vi "Write_All_Channels_to_Month_file.vi"(0 "Current Time":dbl, 1 "Channel Names":string[](array[string]), 2 "Channel Values":string[](array[string]), 3 "Comments":string[](array[string])) -> (7 "File Updated?":bool)   [LabVIEW 2020]
uses:
  Anemometry/Anemometry Sub Vis/Globals/Preference_global.vi
  Anemometry/Anemometry Sub Vis/Globals/Constants_global.vi
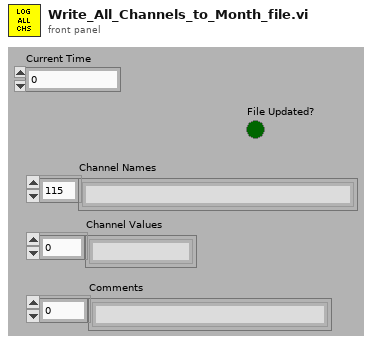
[diagram p1: front panel]
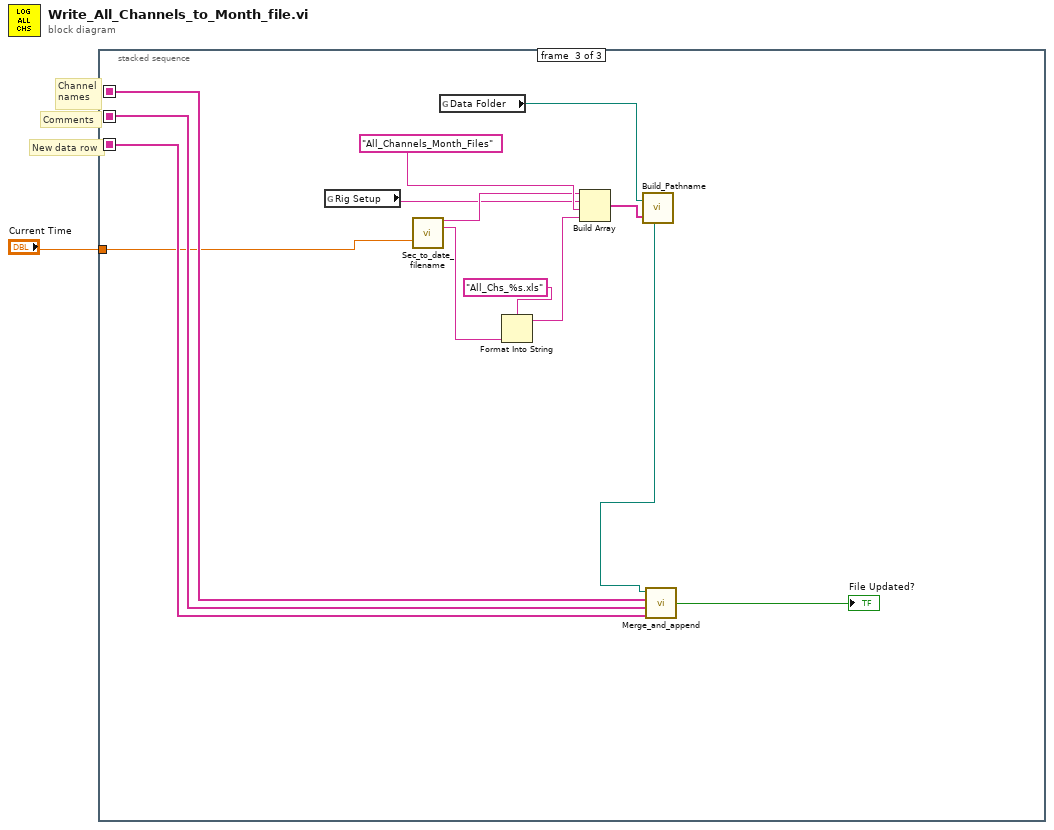
[diagram p0: block diagram]
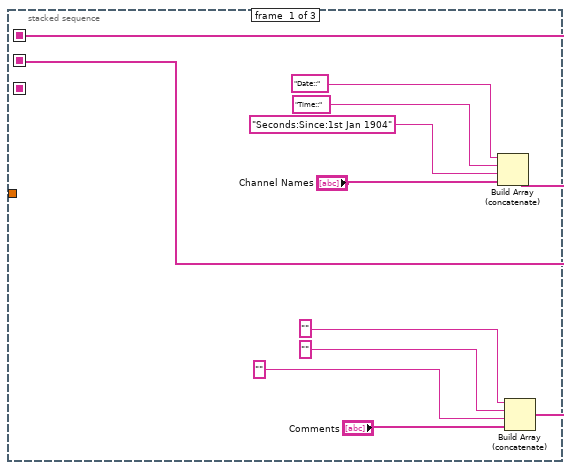
[diagram p2: hidden frame]
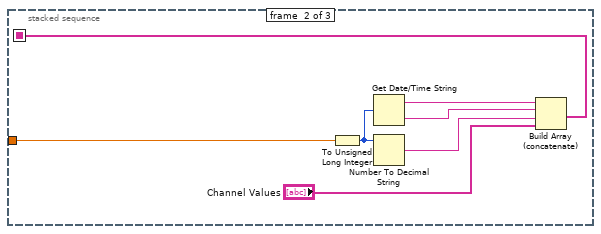
[diagram p3: hidden frame]
diagram:
  # "Comments"
  # "New data row"
  # "Channel\nnames"
  n1 = stacked-sequence {
    seq-local: [w8 _ _] -> [_ _ w32]
    seq-local: [_ w14 _] -> [_ _ w30]
    seq-local: [w4 _ _] -> [_ _ w31]
    tunnel: "Current Time" -> [_ w13 w22]
    frame #0 {
      n2 = Build Array (concatenate)("Date::", "Time::", "Seconds:Since:1st Jan 1904", "Channel Names") -> (w8:string[])
      n3 = Build Array (concatenate)("", "", "", "Comments") -> (w4:string[])
    }
    frame #1 {
      n4 = To Unsigned Long Integer(number=w13) -> (unsigned 32bit integer=w15:u32)
      n5 = Get Date/Time String(seconds (now)=w15) -> (date string=w18:string, time string=w17:string)  [unwired: 2 out]
      n6 = Number To Decimal String(number=w15) -> (decimal integer string=w16:string)  [unwired: 1 out]
      n7 = Build Array (concatenate)(w18, w17, w16, "Channel Values") -> (w14:string[])
    }
    frame #2 {
      n8 = global read "Preference_global.vi" "Rig Setup"() -> (w26:string)
      n9 = call "Sec_to_date_filename.vi"("ss1904"=w22) -> ("YYYY"=w27:string, "mm-YYYY"=w19:string)  [unwired: 5 in, 8 out]
      n10 = global read "Constants_global.vi" "Data Folder"() -> (w25:path)
      n11 = Format Into String(format string="All_Chs_%s.xls", w19) -> (resulting string=w20:string)  [unwired: 2 in, 1 out]
      n12 = Build Array(w27, w26, "All_Channels_Month_Files" ("Input Element"), w20) -> (w24:string[])
      n13 = call "Build_Pathname.vi"("PathElements"=w24, "PathnameIn"=w25) -> ("AppendedPath"=w23:path)
      n14 = call "Merge_and_append.vi"("New Row"=w30, "Comments"=w31, "Channel Names"=w32, "Path name"=w23) -> ("File Updated?"=→"File Updated?":bool)
    }
  }
